vi "UDP 클라01.vi"() -> ()   [LabVIEW 2018]
uses:
  <vilib>/Utility/tcp.llb/UDP Multicast Read-Only Open.vi
panel:
  out "데이터 출력":string
  in  "정지":bool
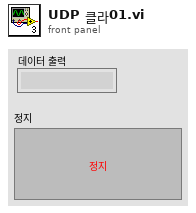
[diagram p1: front panel]
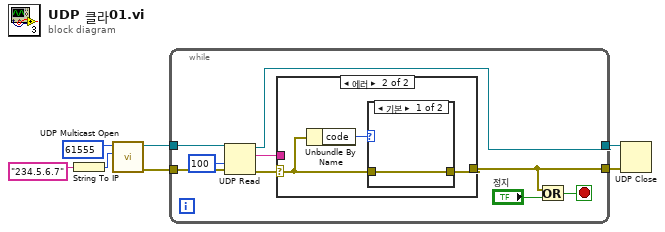
[diagram p0: block diagram]
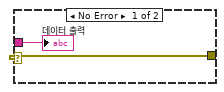
[diagram p2: hidden frame]
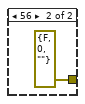
[diagram p3: hidden frame]
diagram:
  n1 = String To IP(1:"234.5.6.7" ("이름")) -> (0:w1:u32)
  n2 = call-poly <vilib>:"UDP Multicast Open.vi"("multicast addr"=w1, "port"=u16 61555 ("포트")) -> ("error out"=w5:errorcluster, "connection ID"=w7:refnum<k16>)  [unwired: 7 in, 1 out]
  n3 = while {
    tunnel: w7 -> [w12]
    tunnel: [w11] -> w6
    tunnel: w5 -> [w16]
    tunnel: [w13] -> w4
    stop <- w15 stop-if-true
    n4 = UDP Read(connection ID=w12, timeout ms (25000)=100 ("타임아웃 ms (25000)"), 8:w16) -> (data out=w10:string, error out=w14:errorcluster, 3:w11:refnum<k16>)  [unwired: 1 in, 2 out]
    n5 = case shown="에러" w14 {
      selector: w14 -> [w18 w19]
      tunnel: [w18 w20] -> w13
      tunnel: w10 -> [w17 _]
      frame No Error {
        "데이터 출력" <- w17
      }
      frame Error {
        n6 = Unbundle By Name(w19) -> ("code"=w21:i32)
        n7 = case shown="기본" w21 {
          tunnel: [w22 errorcluster {"status"=FALSE, "code"=0, "source"=""} ("에러 상수")] -> w20
          tunnel: w19 -> [w22 _]
          frame Default {
          }
          frame 56 {
          }
        }
      }
    }
    n8 = Or(x=w13, y="정지") -> (x .or. y?=w15:bool)
  }
  n9 = UDP Close(connection ID=w6, 8:w4) -> ()  [unwired: 2 out]
